vi "CAN_Write_Read Old.vi"(5 "Read In":refnum<k21>, 6 "Model":string, 8 "CAN frame":T1 {"payload" format="%x"; "timestamp" format="%<%.7X\n%x>T"; "type" items=["CAN Data"=0, "CAN Remote"=1, "CAN Bus Error"=2, "CAN 2.0 Data"=8, "CAN FD Data"=16, "CAN FD+BRS Data"=24, "J1939 Data"=192, "Delay"=224, "Log Trigger"=225, "Start Trigger"=226]; "identifier" format="%x"}, 9 "Write In":refnum<k21>) -> (0 "Error Out":errorcluster, 1 "cluster":T3 {"data[0]"."payload" format="%x"; "data[0]"."timestamp" format="%<%.7X\n%x>T"; "data[0]"."type" items=["CAN Data"=0, "CAN Remote"=1, "CAN Bus Error"=2, "CAN 2.0 Data"=8, "CAN FD Data"=16, "CAN FD+BRS Data"=24, "J1939 Data"=192, "Delay"=224, "Log Trigger"=225, "Start Trigger"=226]; "data[0]"."identifier" format="%x"; "data[1]"."payload" format="%x"; "data[1]"."timestamp" format="%<%.7X\n%x>T"; "data[1]"."type" items=["CAN Data"=0, "CAN Remote"=1, "CAN Bus Error"=2, "CAN 2.0 Data"=8, "CAN FD Data"=16, "CAN FD+BRS Data"=24, "J1939 Data"=192, "Delay"=224, "Log Trigger"=225, "Start Trigger"=226]; "data[1]"."identifier" format="%x"; "data[2]"."payload" format="%x"; "data[2]"."timestamp" format="%<%.7X\n%x>T"; "data[2]"."type" items=["CAN Data"=0, "CAN Remote"=1, "CAN Bus Error"=2, "CAN 2.0 Data"=8, "CAN FD Data"=16, "CAN FD+BRS Data"=24, "J1939 Data"=192, "Delay"=224, "Log Trigger"=225, "Start Trigger"=226]; "data[2]"."identifier" format="%x"; "data[3]"."payload" format="%x"; "data[3]"."timestamp" format="%<%.7X\n%x>T"; "data[3]"."type" items=["CAN Data"=0, "CAN Remote"=1, "CAN Bus Error"=2, "CAN 2.0 Data"=8, "CAN FD Data"=16, "CAN FD+BRS Data"=24, "J1939 Data"=192, "Delay"=224, "Log Trigger"=225, "Start Trigger"=226]; "data[3]"."identifier" format="%x"; "data[4]"."payload" format="%x"; "data[4]"."timestamp" format="%<%.7X\n%x>T"; "data[4]"."type" items=["CAN Data"=0, "CAN Remote"=1, "CAN Bus Error"=2, "CAN 2.0 Data"=8, "CAN FD Data"=16, "CAN FD+BRS Data"=24, "J1939 Data"=192, "Delay"=224, "Log Trigger"=225, "Start Trigger"=226]; "data[4]"."identifier" format="%x"; "data[5]"."payload" format="%x"; "data[5]"."timestamp" format="%<%.7X\n%x>T"; "data[5]"."type" items=["CAN Data"=0, "CAN Remote"=1, "CAN Bus Error"=2, "CAN 2.0 Data"=8, "CAN FD Data"=16, "CAN FD+BRS Data"=24, "J1939 Data"=192, "Delay"=224, "Log Trigger"=225, "Start Trigger"=226]; "data[5]"."identifier" format="%x"; "data[6]"."payload" format="%x"; "data[6]"."timestamp" format="%<%.7X\n%x>T"; "data[6]"."type" items=["CAN Data"=0, "CAN Remote"=1, "CAN Bus Error"=2, "CAN 2.0 Data"=8, "CAN FD Data"=16, "CAN FD+BRS Data"=24, "J1939 Data"=192, "Delay"=224, "Log Trigger"=225, "Start Trigger"=226]; "data[6]"."identifier" format="%x"; "data[7]"."payload" format="%x"; "data[7]"."timestamp" format="%<%.7X\n%x>T"; "data[7]"."type" items=["CAN Data"=0, "CAN Remote"=1, "CAN Bus Error"=2, "CAN 2.0 Data"=8, "CAN FD Data"=16, "CAN FD+BRS Data"=24, "J1939 Data"=192, "Delay"=224, "Log Trigger"=225, "Start Trigger"=226]; "data[7]"."identifier" format="%x"; "data[8]"."payload" format="%x"; "data[8]"."timestamp" format="%<%.7X\n%x>T"; "data[8]"."type" items=["CAN Data"=0, "CAN Remote"=1, "CAN Bus Error"=2, "CAN 2.0 Data"=8, "CAN FD Data"=16, "CAN FD+BRS Data"=24, "J1939 Data"=192, "Delay"=224, "Log Trigger"=225, "Start Trigger"=226]; "data[8]"."identifier" format="%x"}, 2 "Write Out":refnum<k21>, 3 "ID Correct?":bool, 4 "Read Out":refnum<k21>)   [LabVIEW 2023]
uses:
  <vilib>/xnet/xnet.llb/XNET Frame CAN.ctl
  <vilib>/xnet/xnet.llb/XNET Frame Type CAN.ctl
panel:
  in  "Error In":errorcluster
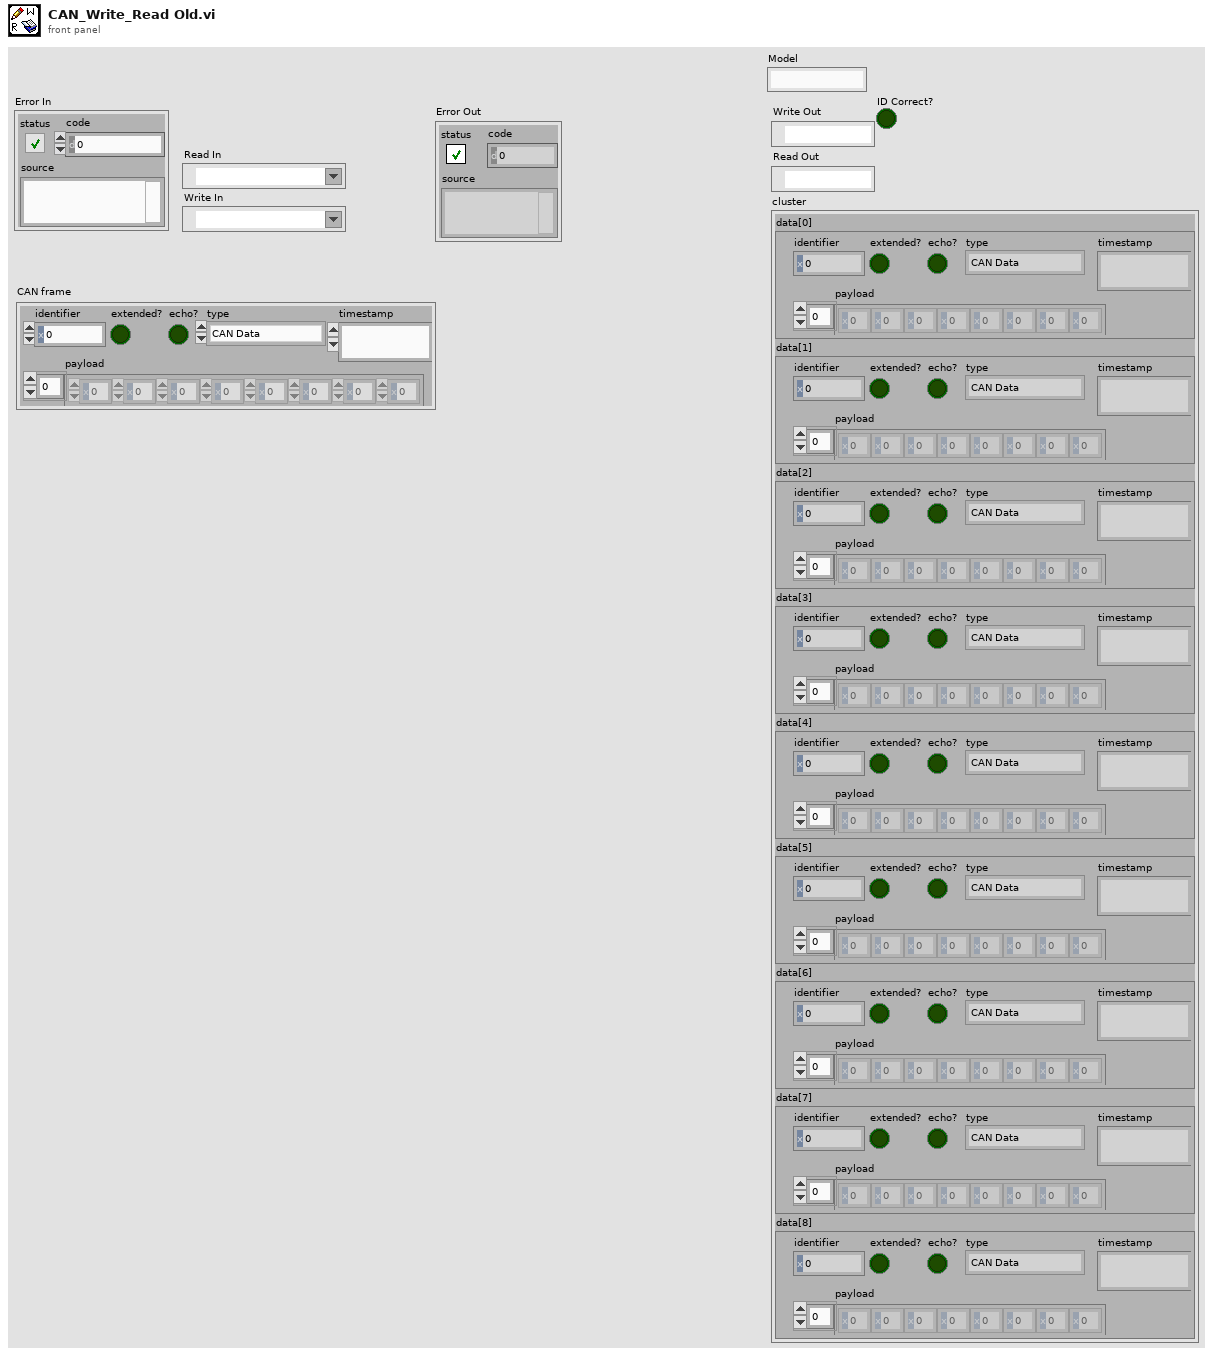
[diagram p1: front panel]
types:
  T1 = typedef "XNET Frame CAN.ctl" = cluster{"timestamp":timestamp, "payload":u8[], "identifier":u32, "type":T2, "extended?":bool, "echo?":bool}
  T2 = typedef "XNET Frame Type CAN.ctl" = u8
  T3 = cluster{"data[0]":T1, "data[1]":T1, "data[2]":T1, "data[3]":T1, "data[4]":T1, "data[5]":T1, "data[6]":T1, "data[7]":T1, "data[8]":T1}
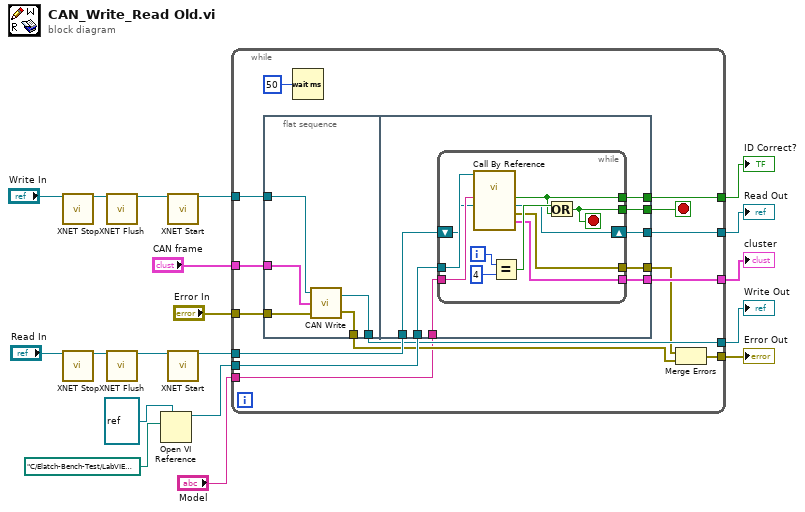
[diagram p0: block diagram]
diagram:
  n1 = call <vilib>:"XNET Stop.vi"("session in"="Write In") -> ("session out"=w12:refnum<k21>)  [unwired: 13 in, 1 out]
  n2 = call <vilib>:"XNET Stop.vi"("session in"="Read In") -> ("session out"=w10:refnum<k21>)  [unwired: 13 in, 1 out]
  n3 = call <vilib>:"XNET Flush.vi"("session in"=w12) -> ("session out"=w11:refnum<k21>)  [unwired: 13 in, 1 out]
  n4 = call <vilib>:"XNET Flush.vi"("session in"=w10) -> ("session out"=w9:refnum<k21>)  [unwired: 13 in, 1 out]
  n5 = Open VI Reference(type specifier VI Refnum (for type only)=refnum<vi> refnum, vi path=path "C:/Elatch-Bench-Test/LabVIEW_VIs/USB 8502/New Version/CAN Read.vi") -> (vi reference=w5:refnum<vi>)  [unwired: 4 in, 1 out]
  n6 = call <vilib>:"XNET Start.vi"("session in"=w11) -> ("session out"=w14:refnum<k21>)  [unwired: 13 in, 1 out]
  n7 = call <vilib>:"XNET Start.vi"("session in"=w9) -> ("session out"=w7:refnum<k21>)  [unwired: 13 in, 1 out]
  n8 = while {
    tunnel: w7 -> [w34]
    tunnel: w5 -> [w33]
    tunnel: [w32] -> w18
    tunnel: "Error In" -> [w31]
    tunnel: w14 -> [w30]
    tunnel: "CAN frame" -> [w29]
    tunnel: [w28] -> w15
    tunnel: [w26] -> w4
    tunnel: [w25] -> w3
    tunnel: [w22] -> w2
    tunnel: "Model" -> [w21]
    stop <- w20 stop-if-true
    n9 = flat-sequence {
      tunnel: w31 -> [w39]
      tunnel: w29 -> [w38]
      tunnel: w30 -> [w37]
      tunnel: [w36] -> w24
      tunnel: [w35] -> w32
      tunnel: w34 -> [w47]
      tunnel: [w46] -> w28
      tunnel: w33 -> [w45]
      tunnel: [w44] -> w26
      tunnel: [w43] -> w25
      tunnel: [w42] -> w23
      tunnel: w21 -> [w41]
      tunnel: [w40] -> w20
      frame #0 {
        n10 = call "CAN Write.vi"("Error In"=w39, "CAN frame"=w38, "Write In"=w37) -> ("Error Out"=w36:errorcluster, "Write Out"=w35:refnum<k21>)
      }
      frame #1 {
        n11 = while {
          tunnel: w45 -> [w55]
          shift-right: [w54] -> w46
          shift-left: w47 -> [w48]
          tunnel: [w51] -> w44
          tunnel: [w53] -> w43
          tunnel: [w52] -> w42
          tunnel: w41 -> [w50]
          tunnel: [w49] -> w40
          i -> [w58]
          stop <- w49 stop-if-true
          n12 = call-by-ref "?"(reference=w55, "Read In"=w48, "Model"=w50) -> ("cluster"=w53:T3, "Error Out"=w52:errorcluster, "Read Out"=w54:refnum<k21>, "ID Correct?"=w51:bool)  [unwired: 3 in, 2 out]
          n13 = Equal?(x=w58, y=4) -> (x = y?=w56:bool)
          n14 = Or(x=w56, y=w51) -> (x .or. y?=w49:bool)
        }
      }
    }
    n15 = Wait (ms)(milliseconds to wait=u32 50) -> ()  [unwired: 1 out]
    n16 = Merge Errors(w23, w24) -> (w22:errorcluster)
  }
  "Write Out" <- w18
  "Error Out" <- w2
  "Read Out" <- w15
  "ID Correct?" <- w4
  "cluster" <- w3
